vi "vector_to_calibration.vi"(8 "Cal data":dbl[][](array[numeric]), 11 "minimum":dbl[](array[numeric])) -> (3 "Calibration out":T1 {"r bias" format="%_3p"; "Ks" format="%#_3p"})   [LabVIEW 2014]
uses:
  calibration.ctl
  mag_globals.vi
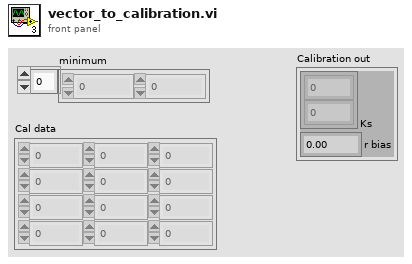
[diagram p1: front panel]
types:
  T1 = typedef "calibration.ctl" = cluster{"Ks":dbl[], "r bias":dbl}
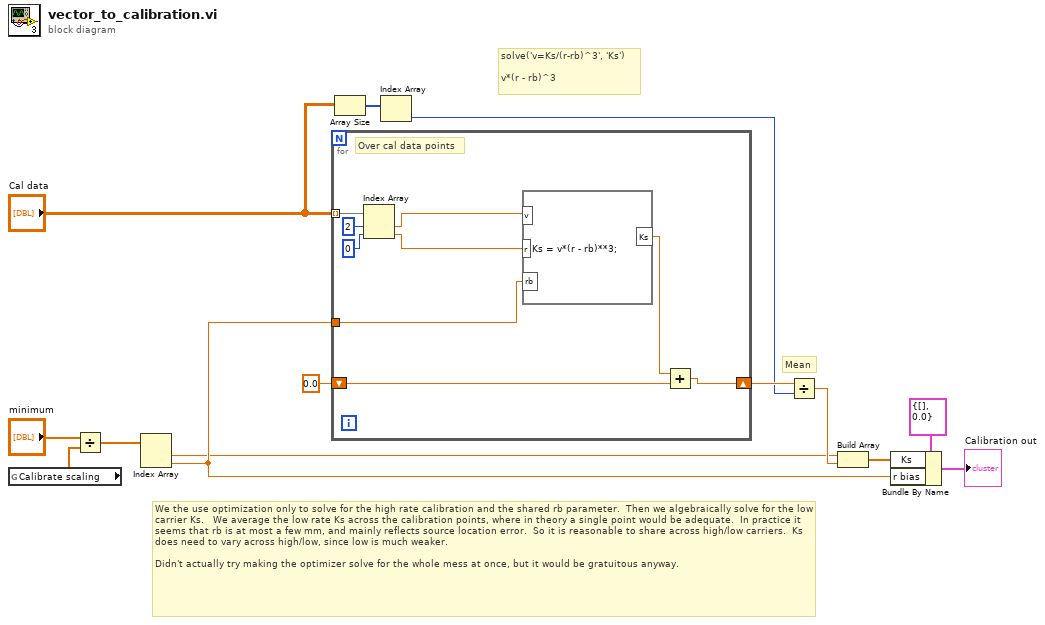
[diagram p0: block diagram]
diagram:
  # "Mean"
  # "solve('v=Ks/(r-rb)^3', 'Ks')\n \nv*(r - rb)^3"
  # "We the use optimization only to solve for the high rate calibration and the shared rb parameter.  Then we algebraically solve for the low carrier Ks.   We average the low rate Ks across the calibration points, where in theory a single point would be adequate.  In practice it seems that rb is at most a few mm, and mainly reflects source location error.  So it is reasonable to share across high/low carriers.  Ks does need to vary across high/low, since low is much weaker.\n\nDidn't actually try making the optimizer solve for the whole mess at once, but it would be gratuitous anyway."
  n1 = global read "mag_globals.vi" "Calibrate scaling"() -> (w13:dbl[])
  n2 = Divide(x="minimum", y=w13) -> (x/y=w9:dbl[])
  n3 = Index Array(array=w9) -> (element #1=w2:dbl, element #2=w8:dbl)  [unwired: 2 in]
  n4 = for {
    tunnel: "Cal data" -> [w20] mode=indexing
    shift-right: [w22] -> w6
    shift-left: 0.0 -> [w23]
    tunnel: w8 -> [w21]
    # "Over cal data points"
    n5 = Index Array(array=w20, index #1=2 ("index"), index #2=0 ("index")) -> (element #1=w16:dbl, element #2=w17:dbl)
    n6 = formula code="Ks = v*(r - rb)**3;"("v"=w16, "r"=w17, "rb"=w21) -> ("Ks"=w15:dbl)
    n7 = Add(x=w15, y=w23) -> (x+y=w22:dbl)
  }
  n8 = Array Size(array="Cal data") -> (size(s)=w7:i32[])
  n9 = Index Array(array=w7) -> (element=w5:i32)  [unwired: 1 in]
  n10 = Divide(x=w6, y=w5) -> (x/y=w4:dbl)
  n11 = Build Array(w2, w4) -> (w1:dbl[])
  n12 = Bundle By Name(cluster=T1 {"Ks"=[], "r bias"=0.0} ("Calibration out"), "Ks"=w1, "r bias"=w8) -> (→"Calibration out":T1)
